vi "SettingsVI.vi"(1 "Config MAIN":refnum<class "Config.lvclass">, 2 "user event":refnum<user-event>) -> ()   [LabVIEW 2015]
uses:
  Classes/Config/Config.lvclass
  Clusters-def/SERVER-Commands.ctl
  globalVarII.vi
  Classes/Control/Control-Server/Control-Server.lvclass
panel:
  out "error out":errorcluster
  in  "Save":bool
  in  "Configuration":string
  in  "stop":bool
  in  "Settings":i32(listbox)
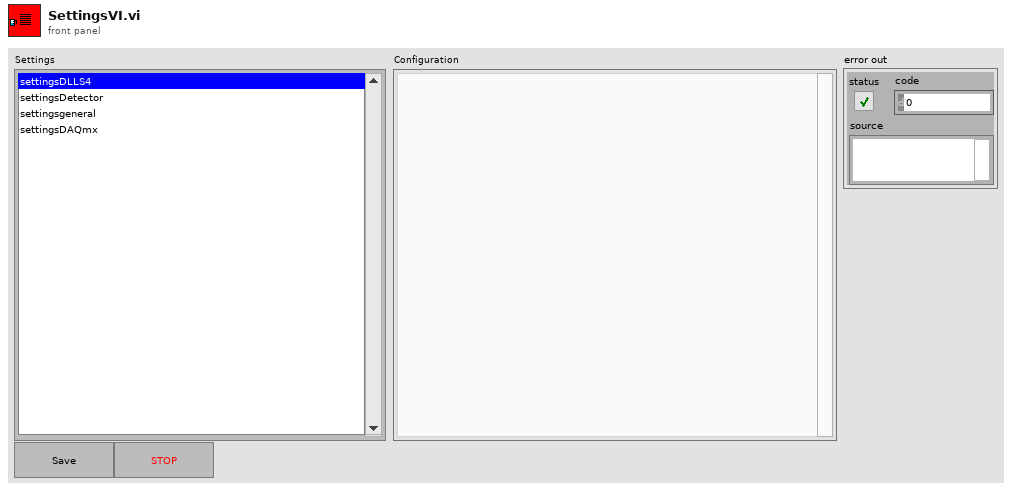
[diagram p1: front panel]
types:
  T1 = typedef "Control-Server.lvclass/SERVER-Commands.ctl" = string
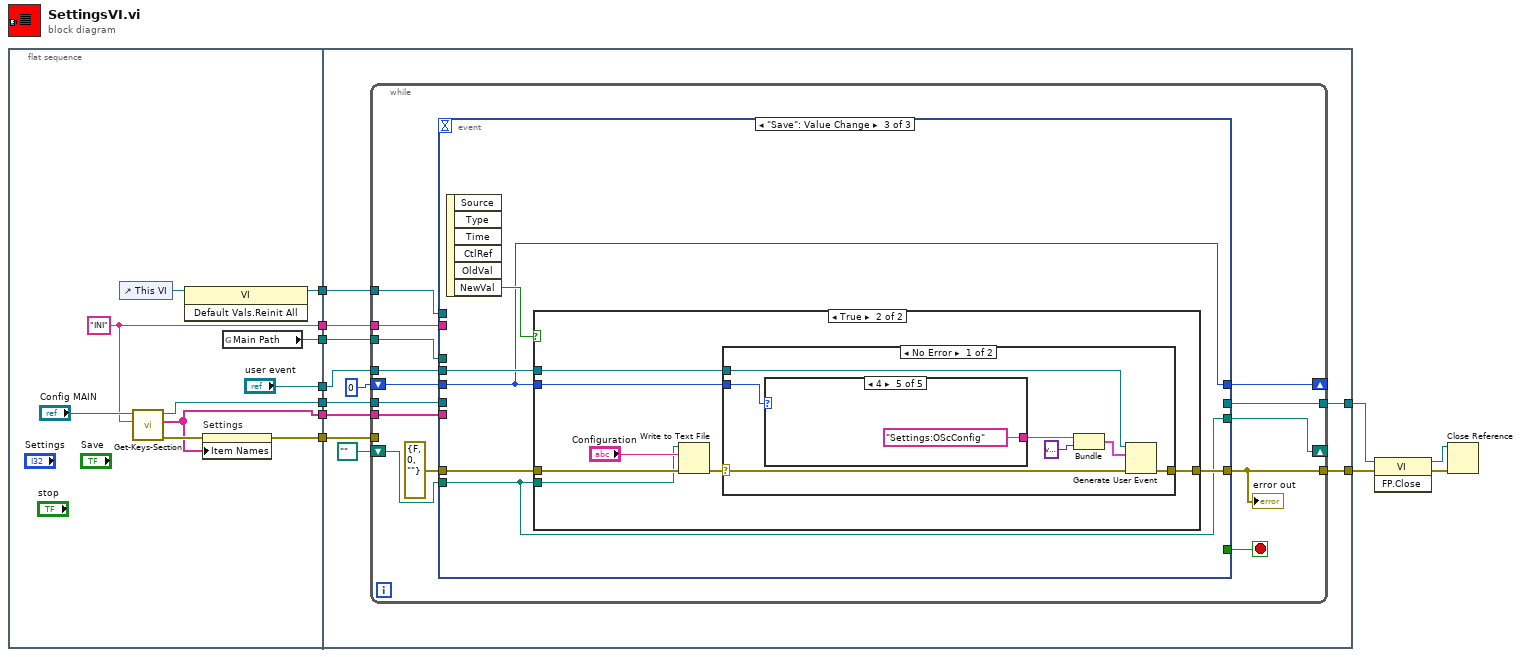
[diagram p0: block diagram]
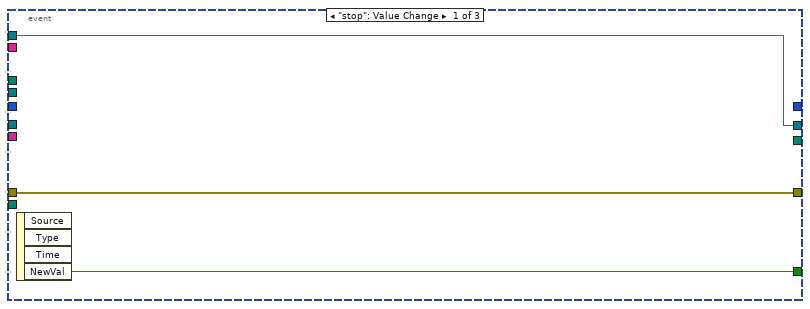
[diagram p2: hidden frame]
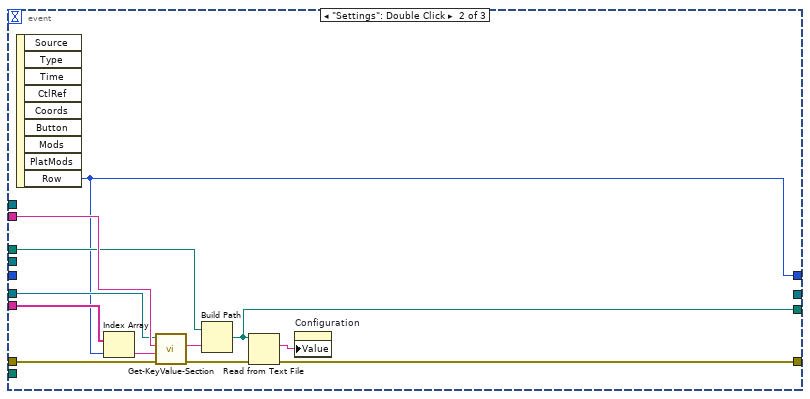
[diagram p3: hidden frame]
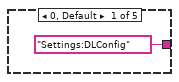
[diagram p5: hidden frame]
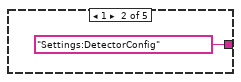
[diagram p6: hidden frame]
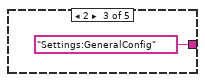
[diagram p7: hidden frame]
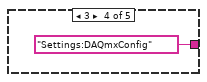
[diagram p8: hidden frame]
diagram:
  n1 = flat-sequence {
    tunnel: [w19] -> w11
    tunnel: [w18] -> w10
    tunnel: [w17] -> w9
    tunnel: [w16] -> w8
    tunnel: [w15] -> w7
    tunnel: [w13] -> w6
    tunnel: ["user event"] -> w5
    tunnel: w11 -> [w32]
    tunnel: w10 -> [w31]
    tunnel: w9 -> [w30]
    tunnel: w8 -> [w29]
    tunnel: w7 -> [w28]
    tunnel: w6 -> [w27]
    tunnel: [w26] -> w3
    tunnel: w5 -> [w25]
    tunnel: [w22] -> w2
    frame #0 {
      w18 = "INI" ("Section")
      n2 = control-ref of="This VI"() -> (w14:refnum<vi>)
      n3 = call-dynamic "Get-Keys-Section.vi"("Section"=w18, "Config in"="Config MAIN") -> ("error out"=w20:errorcluster, "Keys"=w19:string[], "Config out"=w17:refnum<class "Config.lvclass">)  [unwired: 7 in]
      n4 = invoke class="VI" method="Default Vals.Reinit All"(reference=w14) -> (reference out=w13:refnum<vi>)  [unwired: 2 in, 2 out]
      n5 = property on="Settings" class="LstBox (strict)"(error in=w20, "Item Names"=w19) -> (error out=w16:errorcluster)  [unwired: 1 in, 1 out]
      n6 = global read "globalVarII.vi" "Main Path"() -> (w15:path)
    }
    frame #1 {
      n7 = while {
        tunnel: w32 -> [w46]
        tunnel: w31 -> [w45]
        tunnel: w30 -> [w44]
        tunnel: w29 -> [_]
        tunnel: w28 -> [w43]
        tunnel: w27 -> [w40]
        tunnel: [w39] -> w26
        tunnel: w25 -> [w38]
        shift-right: [w37] -> _
        shift-left: 0 -> [w36]
        shift-right: [w35] -> _
        shift-left: path "" ("Main Path") -> [w34]
        tunnel: [w33] -> w22
        stop <- w41 stop-if-true
        n8 = event shown="[2] \"Save\": Value Change" {
          selector: _ -> [_ _ _]
          dyn-events: _ -> [_ _ _]
          timeout: _ -> [_ _ _]
          tunnel: w46 -> [_ w61 _]
          tunnel: w45 -> [_ w59 _]
          tunnel: w44 -> [_ w58 _]
          tunnel: errorcluster {"status"=FALSE, "code"=0, "source"=""} ("error out") -> [w47 w57 w64]
          tunnel: w43 -> [_ w56 _]
          tunnel: [w47 w53 w67] -> w33
          tunnel: [w49 _ _] -> w41
          tunnel: w40 -> [w48 _ _]
          tunnel: [w48 _ _] -> w39
          tunnel: w38 -> [_ _ w66]
          tunnel: [_ w52 w62] -> w37
          tunnel: w36 -> [_ _ w62]
          tunnel: [_ w51 w63] -> w35
          tunnel: w34 -> [_ _ w63]
          event "stop": Value Change {
            n9 = event-data() -> ("NewVal"=w49:bool)  [unwired: 1 in, 3 out]
          }
          event "Settings": Double Click {
            n10 = event-data() -> ("Row"=w52:i32)  [unwired: 1 in, 8 out]
            n11 = Index Array(array=w61, index=w52) -> (element=w60:string)
            n12 = call-dynamic "Get-KeyValue-Section.vi"("error in (no error)"=w57, "Key"=w60, "Section"=w59, "Config in"=w58) -> ("error out"=w54:errorcluster, "Value"=w55:string)  [unwired: 5 in, 1 out]
            n13 = Build Path(base path=w56, name or relative path=w55) -> (appended path=w51:path)
            n14 = Read from Text File(file (use dialog)=w51, error in=w54) -> (text=w50:string, error out=w53:errorcluster)  [unwired: 2 in, 2 out]
            n15 = property on="Configuration" class="Str"("Value"=w50) -> ()  [unwired: 2 in, 2 out]
          }
          event "Save": Value Change {
            n16 = event-data() -> ("NewVal"=w65:bool)  [unwired: 1 in, 5 out]
            n17 = case shown="True" w65 {
              tunnel: [w68 w75] -> w67
              tunnel: w66 -> [_ w74]
              tunnel: w62 -> [_ w73]
              tunnel: w64 -> [w68 w71]
              tunnel: w63 -> [_ w69]
              frame False {
              }
              frame True {
                n18 = Write to Text File(file (use dialog)=w69, text="Configuration", error in=w71) -> (error out=w70:errorcluster)  [unwired: 1 in, 2 out]
                n19 = case shown="No Error" w70 {
                  selector: w70 -> [w76 w88]
                  tunnel: [w82 w88] -> w75
                  tunnel: w74 -> [w81 _]
                  tunnel: w73 -> [w77 _]
                  frame No Error {
                    n20 = case shown="4" w77 {
                      tunnel: [T1 "Settings:DLConfig" ("Commands") T1 "Settings:DetectorConfig" ("Commands") T1 "Settings:GeneralConfig" ("Commands") T1 "Settings:DAQmxConfig" ("Commands") T1 "Settings:OScConfig" ("Commands")] -> w80
                      frame 0, Default {
                      }
                      frame 1 {
                      }
                      frame 2 {
                      }
                      frame 3 {
                      }
                      frame 4 {
                      }
                    }
                    n21 = Bundle("Commands"=w80, variant) -> (w78:cluster{"Commands":T1, variant})  [unwired: 1 in]
                    n22 = Generate User Event(user event=w81, event data cluster=w78, error in=w76) -> (error out=w82:errorcluster)  [unwired: 1 in, 1 out]
                  }
                  frame Error {
                  }
                }
              }
            }
          }
        }
        "error out" <- w33
      }
    }
  }
  n23 = invoke class="VI" method="FP.Close"(reference=w3, error in=w2) -> (reference out=w4:refnum<vi>, error out=w1:errorcluster)  [unwired: 1 in, 1 out]
  n24 = Close Reference(reference=w4, error in (no error)=w1) -> ()  [unwired: 1 out]
